vi "getSortOptions.vi"(8 "error in (no error)":errorcluster, 11 "BasicSortedList in":refnum<class "BasicSortedList.lvclass">) -> (0 "error out":errorcluster, 2 "SortOptions":T1, 3 "BasicSortedList out":refnum<class "BasicSortedList.lvclass">)   [LabVIEW 2009, in "BasicSortedList.lvclass"]
doc: "Get whether the sorted list is asceding or decending."
uses:
  BasicSortedList.lvclass
  BasicSortOptions.ctl
  BasicSortedList.lvclass/BasicSortedList.ctl
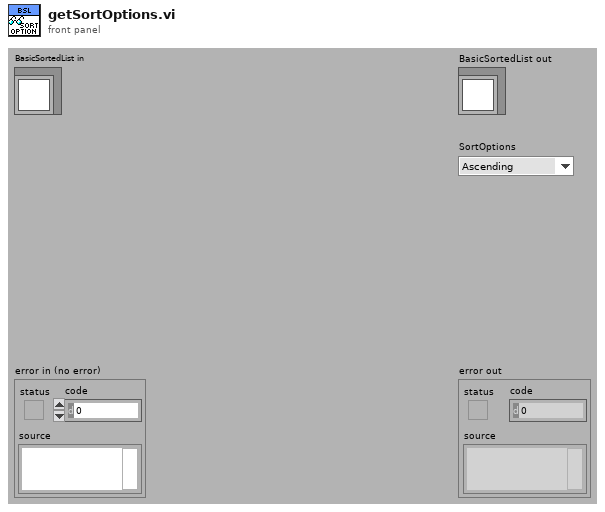
[diagram p1: front panel]
types:
  T1 = typedef "BasicSortedList.lvclass/BasicSortOptions.ctl" = enum16{"Ascending", "Decending"}
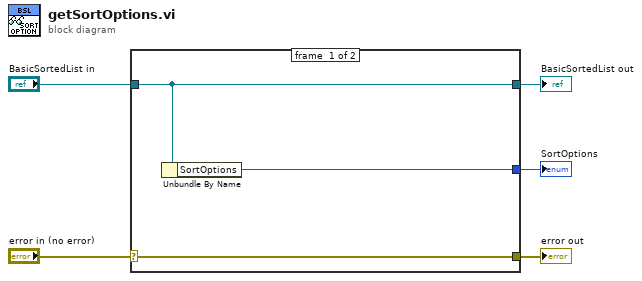
[diagram p0: block diagram]
diagram:
  n1 = case shown="No Error" "error in (no error)" {
    selector: "error in (no error)" -> [w8 w9]
    tunnel: [w8 w9] -> w4
    tunnel: [w7 w10] -> w2
    tunnel: "BasicSortedList in" -> [w7 w10]
    tunnel: [w6 _] -> w1
    frame #0 {
      n2 = Unbundle By Name(w7) -> ("SortOptions"=w6:T1)
    }
    frame #1 {
    }
  }
  "error out" <- w4
  "BasicSortedList out" <- w2
  "SortOptions" <- w1
